vi "Torque2VoltageRot.vi"(11 "torque":dbl) -> (3 "voltage":dbl)   [LabVIEW 2019]
panel:
  # "This Vi calculates from a desired rotational torque the necessary voltage output for the motor."
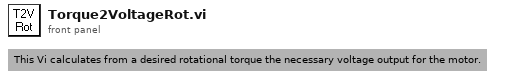
[diagram p1: front panel]
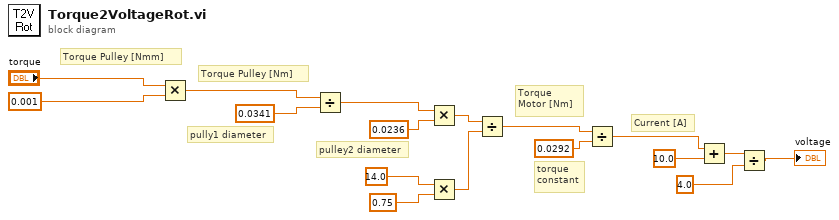
[diagram p0: block diagram]
diagram:
  # "Torque Pulley [Nmm]"
  # "torque \nconstant"
  # "pulley2 diameter"
  # "pully1 diameter"
  # "Torque \nMotor [Nm]"
  # "Torque Pulley [Nm]"
  # "Current [A]"
  n1 = Multiply(x="torque", y=0.001) -> (x*y=w7:dbl)
  n2 = Divide(x=w7, y=0.0341) -> (x/y=w10:dbl)
  n3 = Multiply(x=w10, y=0.0236) -> (x*y=w16:dbl)
  n4 = Multiply(x=14.0 ("value"), y=0.75 ("value")) -> (x*y=w12:dbl)
  n5 = Divide(x=w16, y=w12) -> (x/y=w15:dbl)
  n6 = Divide(x=w15, y=0.0292) -> (x/y=w4:dbl)
  n7 = Add(x=w4, y=10.0) -> (x+y=w3:dbl)
  n8 = Divide(x=w3, y=4.0) -> (x/y=→"voltage":dbl)
